vi "SYRINGPUMPv1.vi"() -> ()   [LabVIEW 2020]
doc: "For Instruments that require characters to be written one at a time. It breaks down the string into individual bytes and transfers one at a time."
panel:
  in  "repeat 3":i32
  in  "repeat 2":i32
  in  "Repeat 1":i32
  in  "pause 1 (ms)":u32=10000
  in  "pause 2 (ms)":u32=10000
  in  "pause 3 (ms)":u32=10000
  in  "VISA resource name 3":refnum<visa-resource-name>
  in  "error in (no error) 3":errorcluster
  out "VISA resource name 3":refnum<visa-resource-name>
  out "error out 3":errorcluster
  out "read buffer 3":string
  out "return count 3":u32
  out "VISA resource name out 3":refnum<visa-resource-name>
  out "output string 3":string
  in  "multi-line string 3":string
  in  "VISA resource name 2":refnum<visa-resource-name>
  in  "error in (no error) 2":errorcluster
  out "VISA resource name 2":refnum<visa-resource-name>
  out "error out 2":errorcluster
  out "read buffer 2":string
  out "return count 2":u32
  out "VISA resource name out 2":refnum<visa-resource-name>
  out "output string 2":string
  in  "multi-line string 2":string
  out "output string 1":string
  out "VISA resource name out 1":refnum<visa-resource-name>
  in  "multi-line string 1":string
  out "return count 1":u32
  out "read buffer 1":string
  out "error out 1":errorcluster
  out "VISA resource name 1":refnum<visa-resource-name>
  in  "error in (no error) 1":errorcluster
  in  "VISA resource name 1":refnum<visa-resource-name>
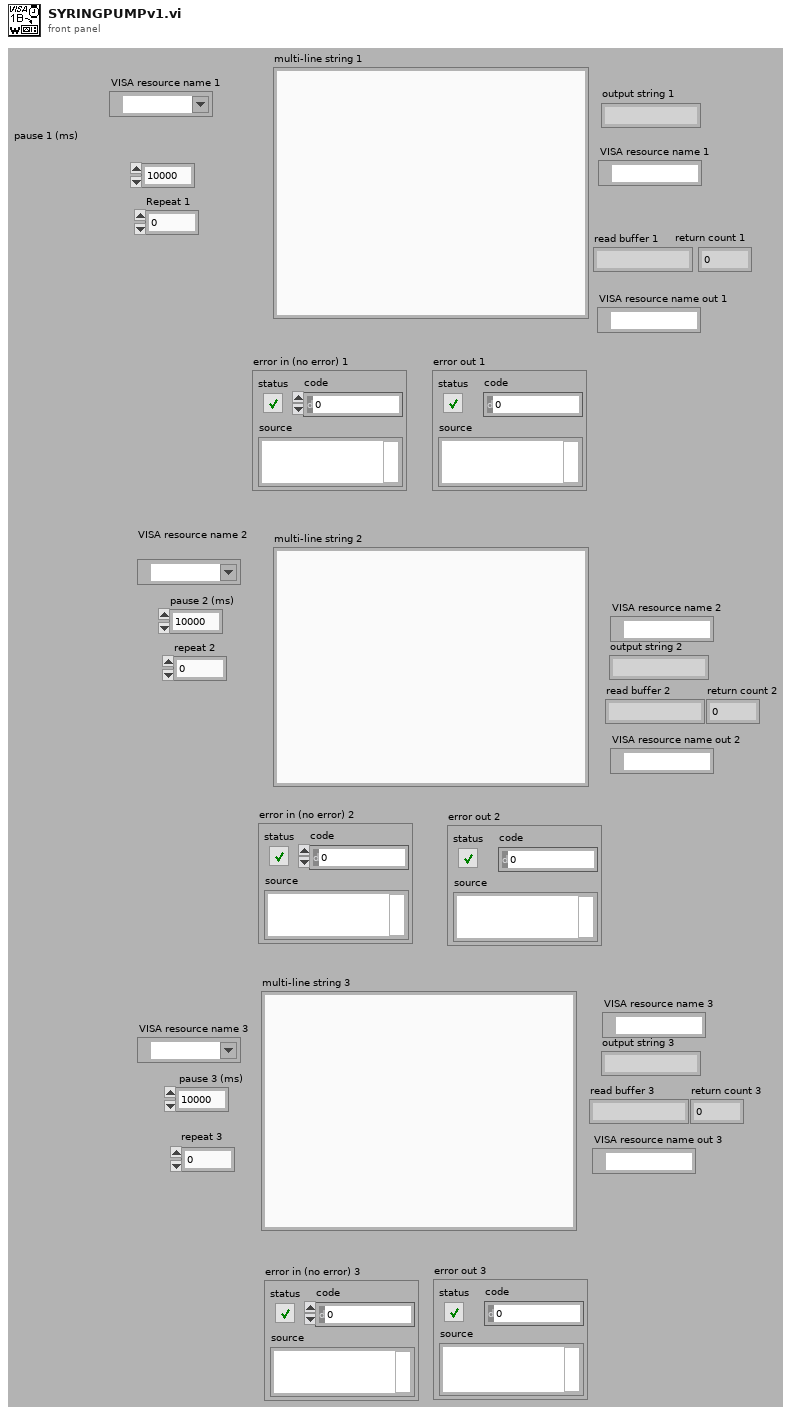
[diagram p1: front panel]
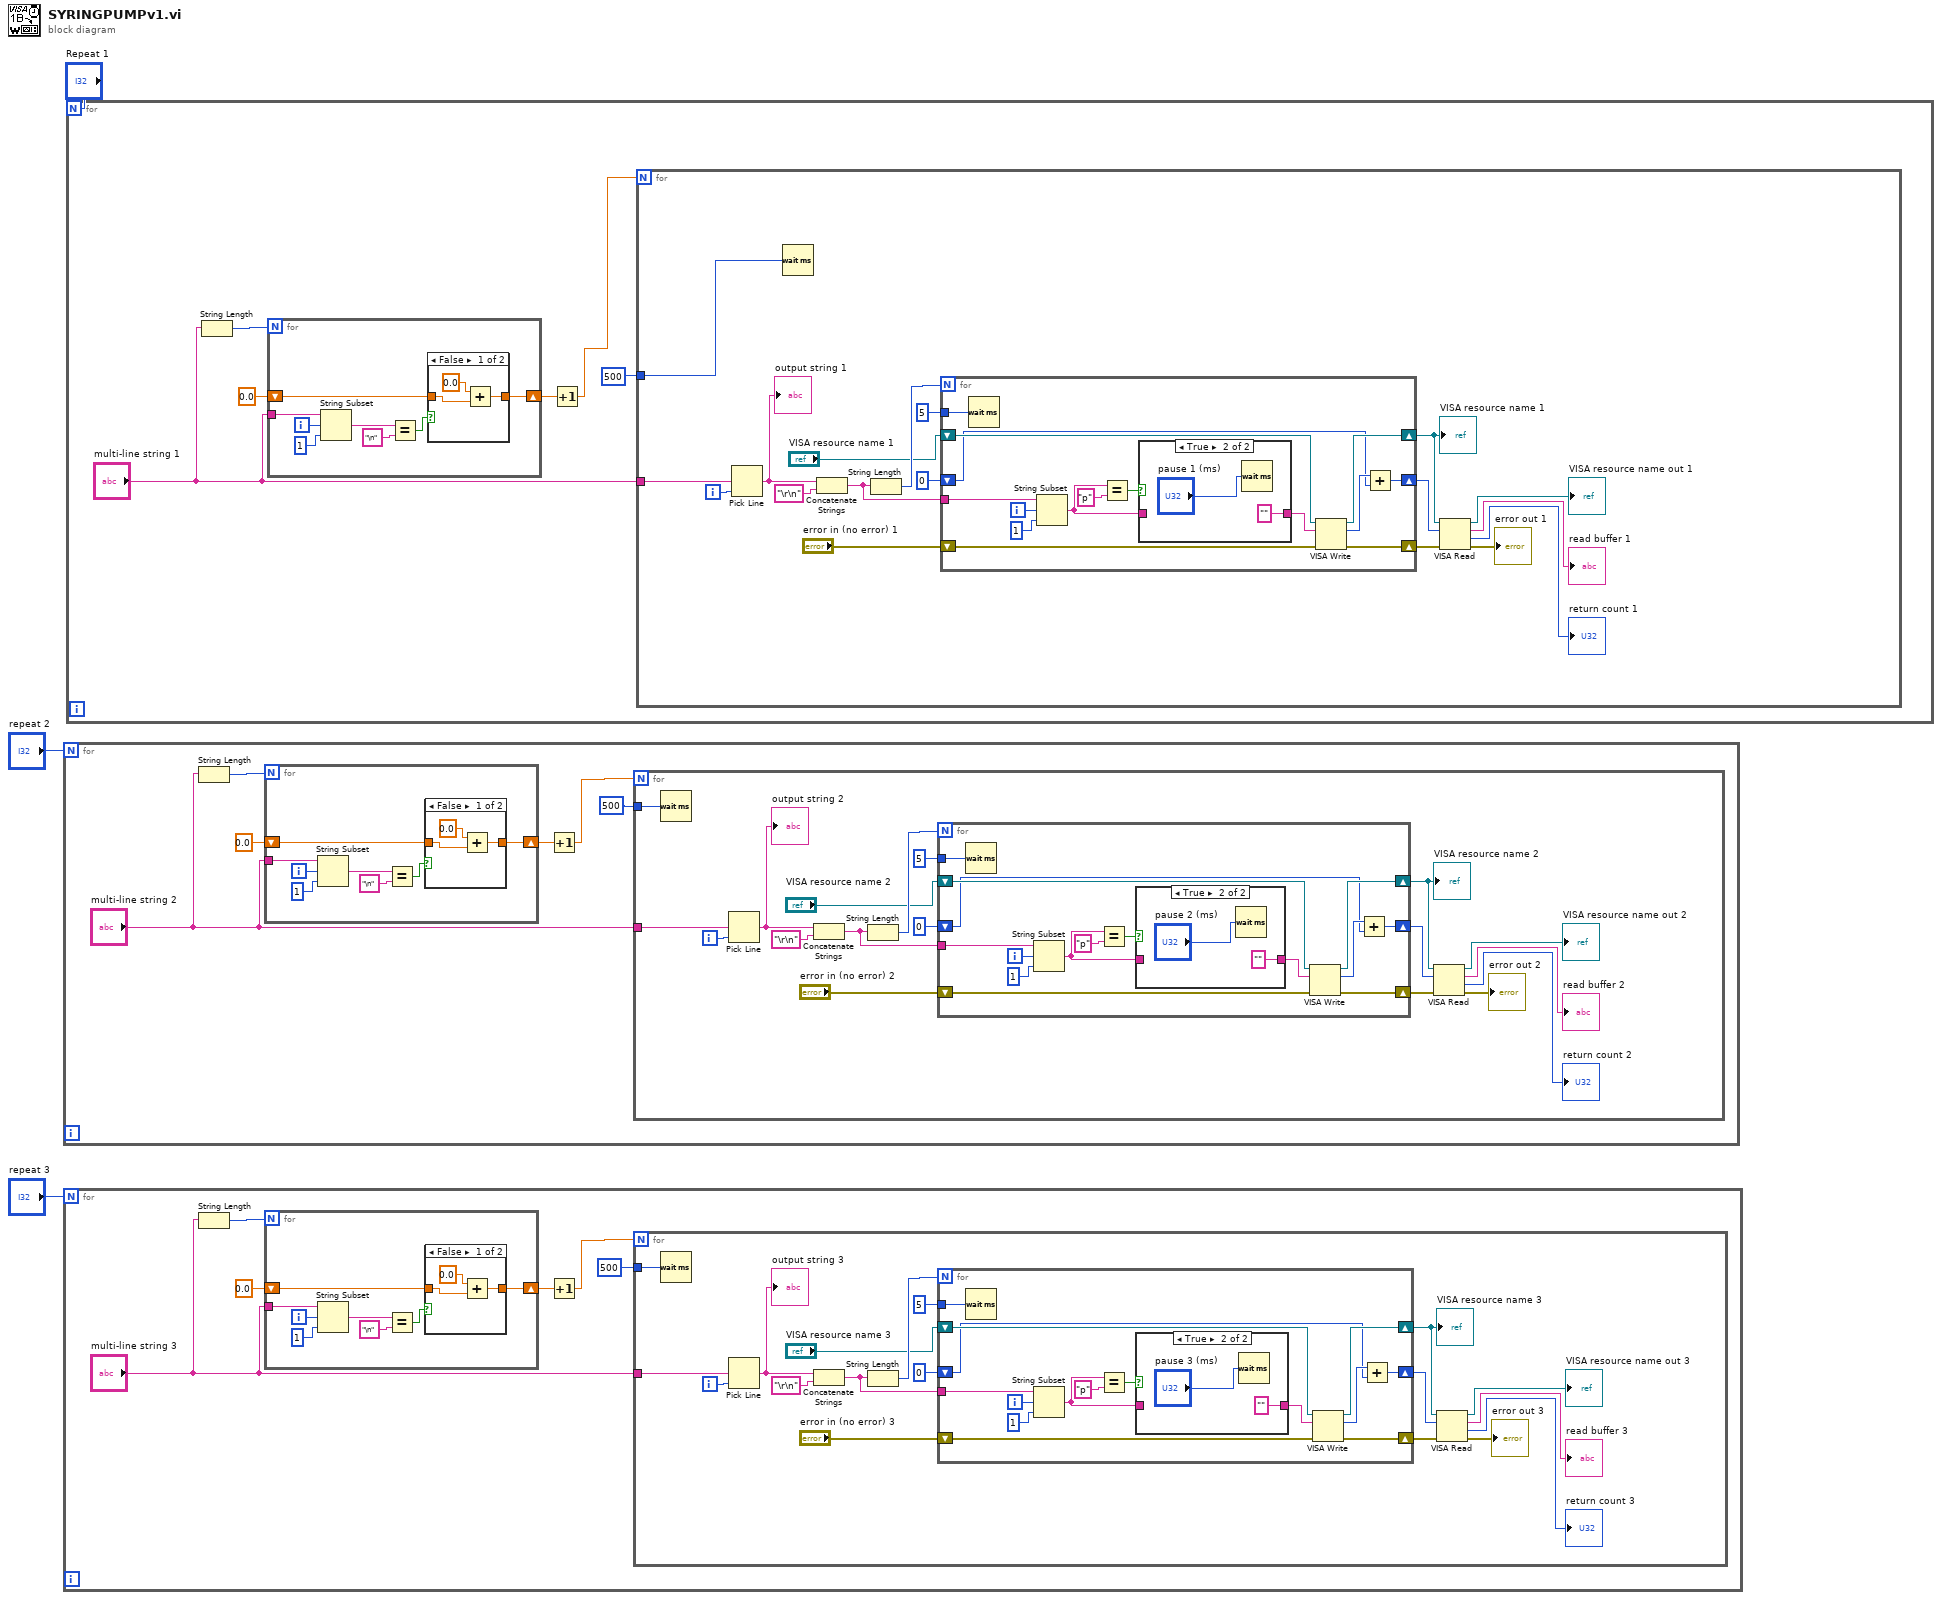
[diagram p0: block diagram]
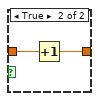
[diagram p2: hidden frame]
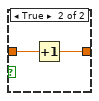
[diagram p4: hidden frame]
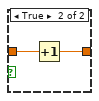
[diagram p6: hidden frame]
diagram:
  n1 = for {
    N: "repeat 2" -> [_]
    n2 = String Length(string="multi-line string 2") -> (length=w7:i32)
    n3 = for {
      N: w7 -> [_]
      tunnel: "multi-line string 2" -> [w15]
      shift-right: [w10] -> w6
      shift-left: 0.0 ("x") -> [w11]
      i -> [w16]
      n4 = String Subset(string=w15, offset (0)=w16, length (rest)=1 ("length (rest)")) -> (substring=w14:string)
      n5 = Equal?(x=w14, y="\n") -> (x = y?=w12:bool)
      n6 = case shown="False" w12 {
        tunnel: w11 -> [w19 w22]
        tunnel: [w18 w21] -> w10
        frame False {
          n7 = Add(x=0.0 ("x+y"), y=w19) -> (x+y=w18:dbl)
        }
        frame True {
          n8 = Increment(x=w22) -> (x+1=w21:dbl)
        }
      }
    }
    n9 = Increment(x=w6) -> (x+1=w5:dbl)
    n10 = for {
      N: w5 -> [_]
      tunnel: "multi-line string 2" -> [w29]
      tunnel: u32 500 ("milliseconds to wait") -> [w23]
      i -> [w28]
      n11 = Wait (ms)(milliseconds to wait=w23) -> ()  [unwired: 1 out]
      n12 = Pick Line(multi-line string=w29, line index=w28) -> (output string=w25:string)  [unwired: 1 in]
      "output string 2" <- w25
      n13 = Concatenate Strings(w25, "\r\n" ("string")) -> (w26:string)
      n14 = String Length(string=w26) -> (length=w40:i32)
      n15 = for {
        N: w40 -> [_]
        tunnel: w26 -> [w55]
        tunnel: u32 5 ("milliseconds to wait 2") -> [w51]
        shift-right: [w49] -> w30
        shift-left: "VISA resource name 2" -> [w53]
        shift-right: [w48] -> w34
        shift-left: "error in (no error) 2" -> [w52]
        shift-right: [w46] -> w35
        shift-left: u32 0 ("y") -> [w47]
        i -> [w54]
        n16 = Wait (ms)(milliseconds to wait=w51) -> ()  [unwired: 1 out]
        n17 = String Subset(string=w55, offset (0)=w54, length (rest)=1 ("length (rest)")) -> (substring=w41:string)
        n18 = Equal?(x=w41, y="p") -> (x = y?=w44:bool)
        n19 = case shown="True" w44 {
          tunnel: [w56 ""] -> w42
          tunnel: w41 -> [w56 _]
          frame False {
          }
          frame True {
            n20 = Wait (ms)(milliseconds to wait="pause 2 (ms)") -> ()  [unwired: 1 out]
          }
        }
        n21 = VISA Write(VISA resource name=w53, write buffer=w42, error in (no error)=w52) -> (VISA resource name out=w49:refnum<visa-resource-name>, return count=w50:u32, error out=w48:errorcluster)
        n22 = Add(x=w50, y=w47) -> (x+y=w46:u32)
      }
      "VISA resource name 2" <- w30
      n23 = VISA Read(VISA resource name=w30, byte count=w35, error in (no error)=w34) -> (VISA resource name out=→"VISA resource name out 2":refnum<visa-resource-name>, read buffer=→"read buffer 2":string, return count=→"return count 2":u32, error out=→"error out 2":errorcluster)
    }
  }
  n24 = for {
    N: "repeat 3" -> [_]
    n25 = String Length(string="multi-line string 3") -> (length=w62:i32)
    n26 = for {
      N: w62 -> [_]
      tunnel: "multi-line string 3" -> [w70]
      shift-right: [w65] -> w61
      shift-left: 0.0 ("x") -> [w66]
      i -> [w71]
      n27 = String Subset(string=w70, offset (0)=w71, length (rest)=1 ("length (rest)")) -> (substring=w69:string)
      n28 = Equal?(x=w69, y="\n") -> (x = y?=w67:bool)
      n29 = case shown="False" w67 {
        tunnel: w66 -> [w74 w77]
        tunnel: [w73 w76] -> w65
        frame False {
          n30 = Add(x=0.0 ("x+y"), y=w74) -> (x+y=w73:dbl)
        }
        frame True {
          n31 = Increment(x=w77) -> (x+1=w76:dbl)
        }
      }
    }
    n32 = Increment(x=w61) -> (x+1=w60:dbl)
    n33 = for {
      N: w60 -> [_]
      tunnel: "multi-line string 3" -> [w84]
      tunnel: u32 500 ("milliseconds to wait") -> [w78]
      i -> [w83]
      n34 = Wait (ms)(milliseconds to wait=w78) -> ()  [unwired: 1 out]
      n35 = Pick Line(multi-line string=w84, line index=w83) -> (output string=w80:string)  [unwired: 1 in]
      "output string 3" <- w80
      n36 = Concatenate Strings(w80, "\r\n" ("string")) -> (w81:string)
      n37 = String Length(string=w81) -> (length=w95:i32)
      n38 = for {
        N: w95 -> [_]
        tunnel: w81 -> [w110]
        tunnel: u32 5 ("milliseconds to wait 3") -> [w106]
        shift-right: [w104] -> w85
        shift-left: "VISA resource name 3" -> [w108]
        shift-right: [w103] -> w89
        shift-left: "error in (no error) 3" -> [w107]
        shift-right: [w101] -> w90
        shift-left: u32 0 ("y") -> [w102]
        i -> [w109]
        n39 = Wait (ms)(milliseconds to wait=w106) -> ()  [unwired: 1 out]
        n40 = String Subset(string=w110, offset (0)=w109, length (rest)=1 ("length (rest)")) -> (substring=w96:string)
        n41 = Equal?(x=w96, y="p") -> (x = y?=w99:bool)
        n42 = case shown="True" w99 {
          tunnel: [w111 ""] -> w97
          tunnel: w96 -> [w111 _]
          frame False {
          }
          frame True {
            n43 = Wait (ms)(milliseconds to wait="pause 3 (ms)") -> ()  [unwired: 1 out]
          }
        }
        n44 = VISA Write(VISA resource name=w108, write buffer=w97, error in (no error)=w107) -> (VISA resource name out=w104:refnum<visa-resource-name>, return count=w105:u32, error out=w103:errorcluster)
        n45 = Add(x=w105, y=w102) -> (x+y=w101:u32)
      }
      "VISA resource name 3" <- w85
      n46 = VISA Read(VISA resource name=w85, byte count=w90, error in (no error)=w89) -> (VISA resource name out=→"VISA resource name out 3":refnum<visa-resource-name>, read buffer=→"read buffer 3":string, return count=→"return count 3":u32, error out=→"error out 3":errorcluster)
    }
  }
  n47 = for {
    N: "Repeat 1" -> [_]
    n48 = String Length(string="multi-line string 1") -> (length=w117:i32)
    n49 = for {
      N: w117 -> [_]
      tunnel: "multi-line string 1" -> [w125]
      shift-right: [w120] -> w116
      shift-left: 0.0 ("x") -> [w121]
      i -> [w126]
      n50 = String Subset(string=w125, offset (0)=w126, length (rest)=1 ("length (rest)")) -> (substring=w124:string)
      n51 = Equal?(x=w124, y="\n") -> (x = y?=w122:bool)
      n52 = case shown="False" w122 {
        tunnel: w121 -> [w129 w132]
        tunnel: [w128 w131] -> w120
        frame False {
          n53 = Add(x=0.0 ("x+y"), y=w129) -> (x+y=w128:dbl)
        }
        frame True {
          n54 = Increment(x=w132) -> (x+1=w131:dbl)
        }
      }
    }
    n55 = Increment(x=w116) -> (x+1=w115:dbl)
    n56 = for {
      N: w115 -> [_]
      tunnel: "multi-line string 1" -> [w139]
      tunnel: u32 500 ("milliseconds to wait") -> [w133]
      i -> [w138]
      n57 = Pick Line(multi-line string=w139, line index=w138) -> (output string=w135:string)  [unwired: 1 in]
      "output string 1" <- w135
      n58 = Wait (ms)(milliseconds to wait=w133) -> ()  [unwired: 1 out]
      n59 = Concatenate Strings(w135, "\r\n" ("string")) -> (w136:string)
      n60 = String Length(string=w136) -> (length=w150:i32)
      n61 = for {
        N: w150 -> [_]
        tunnel: w136 -> [w165]
        tunnel: u32 5 ("milliseconds to wait") -> [w161]
        shift-right: [w159] -> w140
        shift-left: "VISA resource name 1" -> [w163]
        shift-right: [w158] -> w144
        shift-left: "error in (no error) 1" -> [w162]
        shift-right: [w156] -> w145
        shift-left: u32 0 ("y") -> [w157]
        i -> [w164]
        n62 = Wait (ms)(milliseconds to wait=w161) -> ()  [unwired: 1 out]
        n63 = String Subset(string=w165, offset (0)=w164, length (rest)=1 ("length (rest)")) -> (substring=w151:string)
        n64 = Equal?(x=w151, y="p") -> (x = y?=w154:bool)
        n65 = case shown="True" w154 {
          tunnel: [w166 ""] -> w152
          tunnel: w151 -> [w166 _]
          frame False {
          }
          frame True {
            n66 = Wait (ms)(milliseconds to wait="pause 1 (ms)") -> ()  [unwired: 1 out]
          }
        }
        n67 = VISA Write(VISA resource name=w163, write buffer=w152, error in (no error)=w162) -> (VISA resource name out=w159:refnum<visa-resource-name>, return count=w160:u32, error out=w158:errorcluster)
        n68 = Add(x=w160, y=w157) -> (x+y=w156:u32)
      }
      "VISA resource name 1" <- w140
      n69 = VISA Read(VISA resource name=w140, byte count=w145, error in (no error)=w144) -> (VISA resource name out=→"VISA resource name out 1":refnum<visa-resource-name>, read buffer=→"read buffer 1":string, return count=→"return count 1":u32, error out=→"error out 1":errorcluster)
    }
  }
